vi "Connections_FGV.vi"(8 "error in (no error)":errorcluster, 11 "connection string in":string) -> (0 "error out":errorcluster, 3 "connection string out":string)   [LabVIEW 2019, in "LV-Data.PGSQL.lvclass"]
uses:
  LV-Data.PGSQL.lvclass
  PGPASS/PGPASS.lvlib
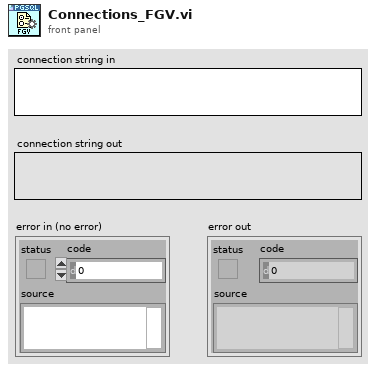
[diagram p1: front panel]
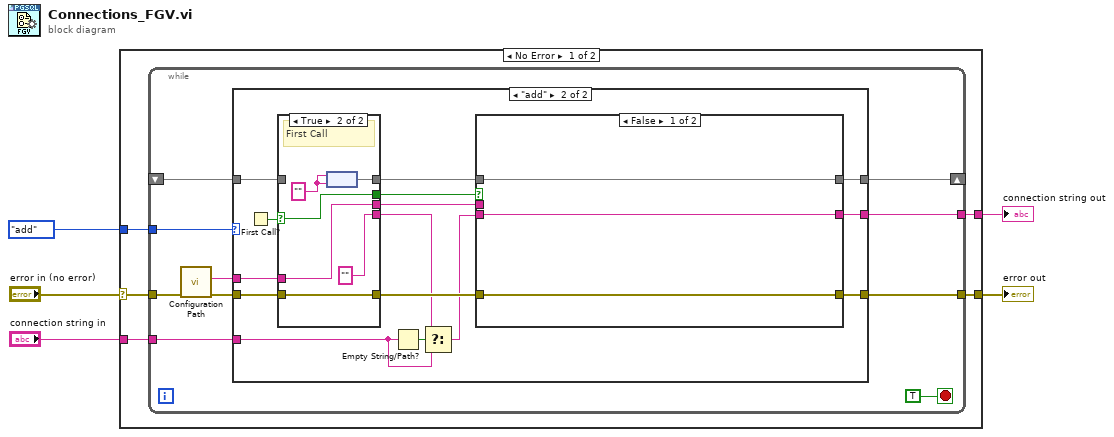
[diagram p0: block diagram]
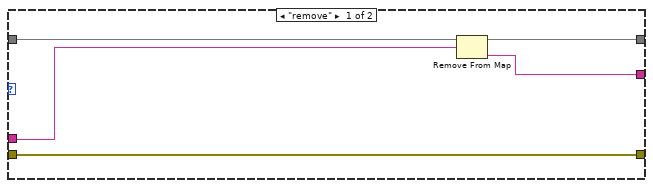
[diagram p2: hidden frame]
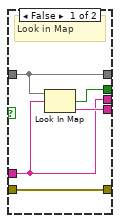
[diagram p3: hidden frame]
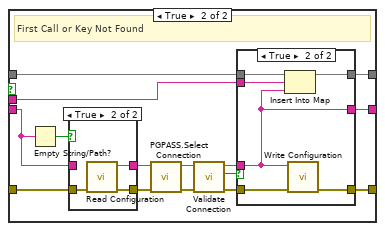
[diagram p4: hidden frame]
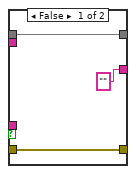
[diagram p6: hidden frame]
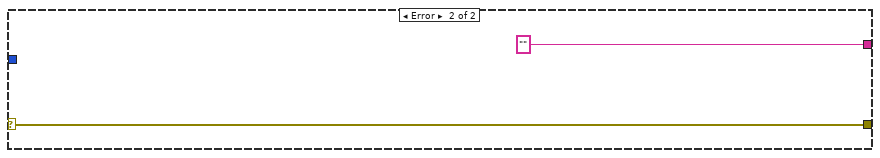
[diagram p7: hidden frame]
diagram:
  n1 = case shown="No Error" "error in (no error)" {
    selector: "error in (no error)" -> [w10 w85]
    tunnel: [w9 w85] -> w5
    tunnel: [w8 "" ("Connection Strings out")] -> w3
    tunnel: "connection string in" -> [w7 _]
    tunnel: enum16{"add", "remove"}."add" ("action") -> [w6 _]
    frame No Error {
      n2 = while {
        shift-right: [w15] -> _
        shift-left: _ -> [w19]
        tunnel: [w14] -> w8
        tunnel: w7 -> [w12]
        tunnel: w6 -> [w11]
        tunnel: w10 -> [w20]
        tunnel: [w13] -> w9
        stop <- TRUE stop-if-true
        n3 = call "Configuration Path.vi"("error in (no error)"=w20) -> ("error out"=w16:errorcluster, "section"=w17:string)  [unwired: 8 in, 1 out]
        n4 = case shown="\"add\"" w11 {
          tunnel: w19 -> [w25 w40]
          tunnel: w17 -> [w24 w39]
          tunnel: w16 -> [w21 w36]
          tunnel: [w23 w33] -> w15
          tunnel: [w22 w32] -> w14
          tunnel: [w21 w30] -> w13
          tunnel: w12 -> [_ w26]
          frame "remove" {
            n5 = Remove From Map(10:w24, 11:w25) -> (1:w22:string, 3:w23:map{string, string})  [unwired: 1 out]
          }
          frame "add" {
            n6 = First Call?() -> (First Call?: T/F=w38:bool)
            n7 = case shown="True" w38 {
              selector: w38 -> [_ w48]
              tunnel: w39 -> [w42 w46]
              tunnel: w40 -> [w45 _]
              tunnel: [w41 w48] -> w37
              tunnel: [w45 w50] -> w34
              tunnel: w36 -> [w44 w49]
              tunnel: [w44 w49] -> w35
              tunnel: [w43 "" ("value")] -> w28
              tunnel: [w42 w46] -> w31
              frame False {
                # "Look in Map"
                n8 = Look In Map(map=w45, key=w42) -> (key not found?=w41:bool, value=w43:string)  [unwired: 1 in]
              }
              frame True {
                w51 = ""
                # "First Call"
                n9 = node(w51, w51) -> (w50:map{string, string})
              }
            }
            n10 = Empty String/Path?(string/path=w26) -> (empty?=w29:bool)
            n11 = Select(t=w28, s=w29, f=w26) -> (s? t:f=w27:string)
            n12 = case shown="False" w37 {
              tunnel: w35 -> [w52 w69]
              tunnel: w27 -> [w54 w55]
              tunnel: w34 -> [w53 w58]
              tunnel: [w53 w63] -> w33
              tunnel: [w54 w57] -> w32
              tunnel: w31 -> [_ w62]
              tunnel: [w52 w59] -> w30
              frame False {
              }
              frame True {
                # "First Call or Key Not Found"
                n13 = Empty String/Path?(string/path=w55) -> (empty?=w56:bool)
                n14 = case shown="True" w56 {
                  tunnel: w69 -> [w71 w74]
                  tunnel: [w71 w73] -> w68
                  tunnel: [w70 w72] -> w67
                  tunnel: w55 -> [w70 _]
                  frame False {
                  }
                  frame True {
                    n15 = call "Read Configuration.vi"("error in (no error)"=w74) -> ("error out"=w73:errorcluster, "connection string"=w72:string)  [unwired: 9 in]
                  }
                }
                n16 = call "PGPASS.Select Connection.vi"("error in"=w68, "search string"=w67) -> ("error out"=w66:errorcluster, "connection string"=w65:string)  [unwired: 8 in]
                n17 = call "Validate Connection.vi"("error in (no error)"=w66, "Connection String in"=w65) -> ("error out"=w60:errorcluster, "OK?"=w64:bool, "Connection String out"=w61:string)  [unwired: 6 in, 1 out]
                n18 = case shown="True" w64 {
                  tunnel: [w77 w82] -> w63
                  tunnel: w62 -> [_ w81]
                  tunnel: w61 -> [_ w78]
                  tunnel: w60 -> [w76 w80]
                  tunnel: [w76 w79] -> w59
                  tunnel: w58 -> [w77 w83]
                  tunnel: ["" ("Connection Strings out") w78] -> w57
                  frame False {
                  }
                  frame True {
                    n19 = Insert Into Map(map in=w83, key=w81, value=w78) -> (map out=w82:map{string, string})  [unwired: 2 out]
                    n20 = call "Write Configuration.vi"("error in (no error)"=w80, "connection string"=w78) -> ("error out"=w79:errorcluster)  [unwired: 9 in]
                  }
                }
              }
            }
          }
        }
      }
    }
    frame Error {
    }
  }
  "error out" <- w5
  "connection string out" <- w3
